vi "Pixel Array Long & Short Axis Length & Aspect Ratio.vi"(8 "error in (no error)":errorcluster, 9 "Direction":cluster{"x":dbl, "y":dbl}, 10 "Center":cluster{"x":sgl, "y":sgl}, 11 "Pixel Coordinates":T1[](array[typedef])) -> (0 "error out":errorcluster, 1 "Aspect Ratio":dbl, 2 "Short Axis Length":dbl, 3 "Long Axis Length":dbl)   [LabVIEW 2021, in "Image.lvlib"]
doc: "Computes the length of the projections of the <B>Pixel Coordinates</B> on the axes formed by the <B>Center</B> and the <B>Direction</B> and its orthogonal direction, and returns the differences between max and min of all coordinates along the two axes, as well as their <B>Aspect Ratio</B>.\n\nThe first difference is interpreted as the <B>Long Axis Length</B> and the second as the <B>Short Axis Length</B> when the center is the barycenter of the cloud of points and the direction is that of the minor or major axis of inertia of the array of pixels."
uses:
  Image.lvlib
  Image Point.ctl
panel:
  # "see the AlliGator License on the block diagram (Ctrl+E or Window:Show Block Diagram)"
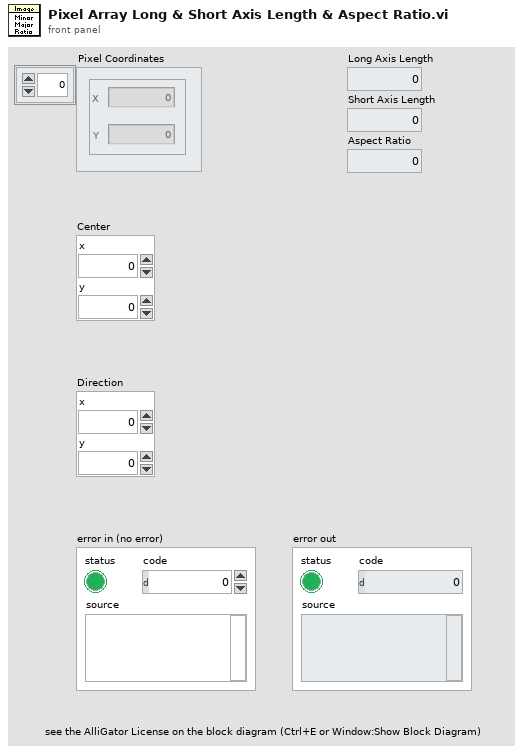
[diagram p1: front panel]
types:
  T1 = typedef "Image.lvlib/Image Point.ctl" = cluster{"X":i32, "Y":i32}
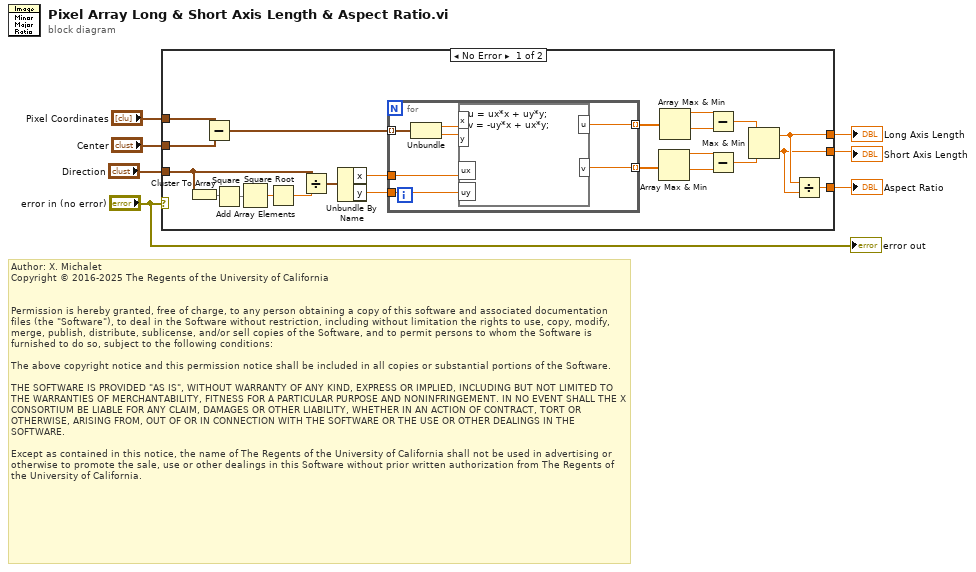
[diagram p0: block diagram]
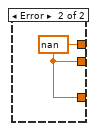
[diagram p2: hidden frame]
diagram:
  # "Author: X. Michalet\nCopyright © 2016-2025 The Regents of the University of California\n \n\nPermission is hereby granted, free of charge, to any person obtaining a copy of this software and associated documentation files (the \"Software\"), to deal in the Software without restriction, including without limitation the rights to use, copy, modify, merge, publish, distribute, sublicense, and/or sell copies of the Software, and to permit persons to whom the Software is furnished to do so, subject to the following conditions:\n\nThe above copyright notice and this permission notice shall be included in all copies or substantial portions of the Software.\n\nTHE SOFTWARE IS PROVIDED \"AS IS\", WITHOUT WARRANTY OF ANY KIND, EXPRESS OR IMPLIED, INCLUDING BUT NOT LIMITED TO THE WARRANTIES OF MERCHANTABILITY, FITNESS FOR A PARTICULAR PURPOSE AND NONINFRINGEMENT. IN NO EVENT SHALL THE X CONSORTIUM BE LIABLE FOR ANY CLAIM, DAMAGES OR OTHER LIABILITY, WHETHER IN AN ACTION OF CONTRACT, TORT OR OTHERWISE, ARISING FROM, OUT OF OR IN CONNECTION WITH THE SOFTWARE OR THE USE OR OTHER DEALINGS IN THE SOFTWARE.\n\nExcept as contained in this notice, the name of The Regents of the University of California shall not be used in advertising or otherwise to promote the sale, use or other dealings in this Software without prior written authorization from The Regents of the University of California."
  n1 = case shown="No Error" "error in (no error)" {
    tunnel: "Pixel Coordinates" -> [w29 _]
    tunnel: "Center" -> [w28 _]
    tunnel: "Direction" -> [w25 _]
    tunnel: [w10 w37] -> w4
    tunnel: [w9 w37] -> w3
    tunnel: [w8 w37] -> w2
    frame No Error {
      n2 = Cluster To Array(cluster=w25) -> (array=w27:dbl[])
      n3 = Subtract(x=w29, y=w28) -> (x-y=w21:cluster{sgl, sgl}[])
      n4 = Square(x=w27) -> (x^2=w26:dbl[])
      n5 = Add Array Elements(numeric array=w26) -> (sum=w23:dbl)
      n6 = Square Root(x=w23) -> (sqrt(x)=w24:dbl)
      n7 = Divide(x=w25, y=w24) -> (x/y=w22:cluster{"x":dbl, "y":dbl})
      n8 = Unbundle By Name(w22) -> ("x"=w20:dbl, "y"=w19:dbl)
      n9 = for {
        tunnel: w21 -> [w36] mode=indexing
        tunnel: w20 -> [w33]
        tunnel: w19 -> [w32]
        tunnel: [w31] -> w18 mode=indexing
        tunnel: [w30] -> w17 mode=indexing
        n10 = Unbundle(w36) -> (w35:sgl, w34:sgl)
        n11 = formula code="u = ux*x + uy*y;\nv = -uy*x + ux*y;"("x"=w35, "y"=w34, "ux"=w33, "uy"=w32) -> ("u"=w31:dbl, "v"=w30:dbl)
      }
      n12 = Array Max & Min(array=w17) -> (max value=w14:dbl, min value=w13:dbl)  [unwired: 2 out]
      n13 = Array Max & Min(array=w18) -> (max value=w16:dbl, min value=w15:dbl)  [unwired: 2 out]
      n14 = Subtract(x=w16, y=w15) -> (x-y=w12:dbl)
      n15 = Subtract(x=w14, y=w13) -> (x-y=w11:dbl)
      n16 = Max & Min(x=w12, y=w11) -> (max(x,y)=w10:dbl, min(x,y)=w9:dbl)
      n17 = Divide(x=w10, y=w9) -> (x/y=w8:dbl)
    }
    frame Error {
      w37 = nan
    }
  }
  "Long Axis Length" <- w4
  "Short Axis Length" <- w3
  "Aspect Ratio" <- w2
  "error out" <- "error in (no error)"
